vi "Configure Comparison Control.vi"(4 "Control Visibility":T1, 7 "Control Refs":T2, 8 "error in (no error)":errorcluster) -> (0 "error out":errorcluster)   [LabVIEW 2018]
uses:
  Comparison Ctrl Refs.ctl
  Comparison Visibility.ctl
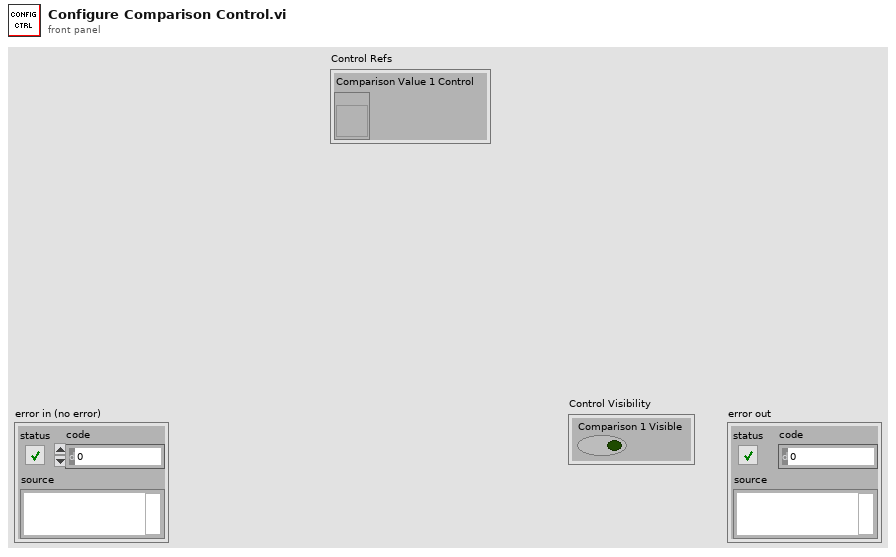
[diagram p1: front panel]
types:
  T1 = typedef "Comparison Visibility.ctl" = cluster{"Comparison 1 Visible":bool}
  T2 = typedef "Comparison Ctrl Refs.ctl" = cluster{"Comparison Value 1 Control":refnum<vi>}
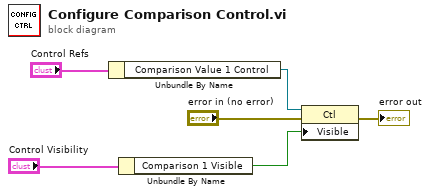
[diagram p0: block diagram]
diagram:
  n1 = Unbundle By Name("Control Refs") -> ("Comparison Value 1 Control"=w3:refnum<vi>)
  n2 = Unbundle By Name("Control Visibility") -> ("Comparison 1 Visible"=w1:bool)
  n3 = property class="Ctl"(reference=w3, error in="error in (no error)", "Visible"=w1) -> (error out=→"error out":errorcluster)  [unwired: 1 out]
